vi "Show UI.vi"(0 "reference in":refnum<class "UI Manager Proxy.lvclass">, 2 "UI Type":T1, 5 "Error In":errorcluster) -> (14 "reference out":refnum<class "UI Manager Proxy.lvclass">, 19 "Error Out":errorcluster)   [LabVIEW 2024, in "UI Manager Proxy.lvclass"]
uses:
  UI Manager Proxy.lvclass
  UIType.ctl
  UI Manager_class/UI Manager.lvclass
  UI Manager Proxy.lvclass/UI Manager Proxy.ctl
panel:
  # "Connector Pane"
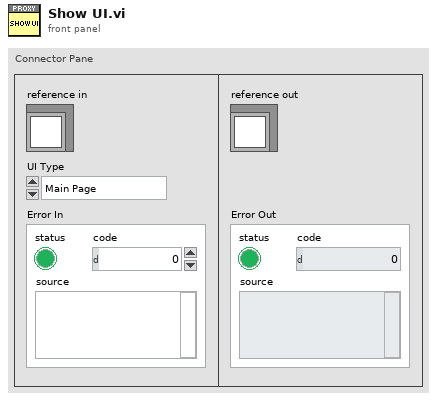
[diagram p1: front panel]
types:
  T1 = typedef "UIType.ctl" = enum16{"Main Page", "Settings Page", "Debugging Page"}
  T2 = typedef "UI Manager Proxy.lvclass/ObjectAttributes.ctl" = cluster{"UI Manager":refnum<class "UI Manager.lvclass">, "UserLevel":T3}
  T3 = typedef "UserLevel.ctl" = enum16{"System Manager", "Admin", "Operator"}
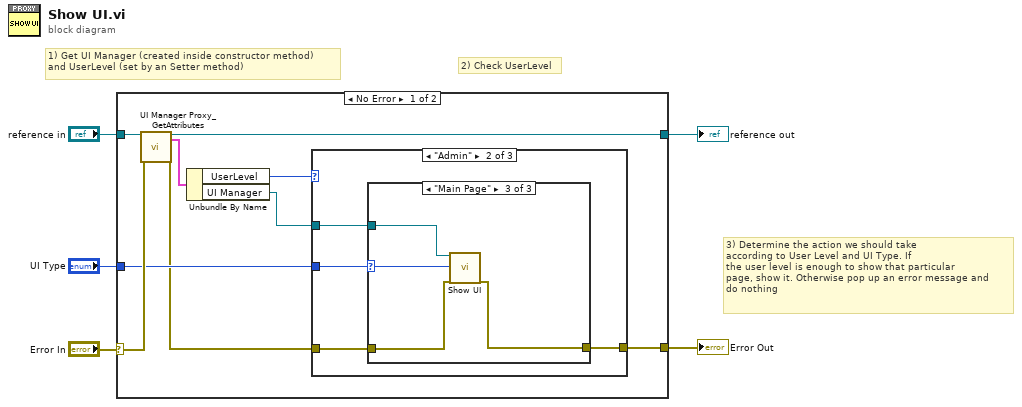
[diagram p0: block diagram]
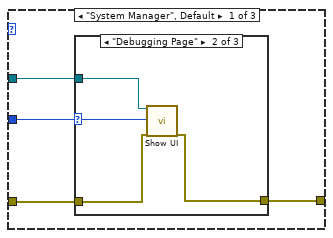
[diagram p2: hidden frame]
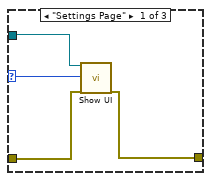
[diagram p3: hidden frame]
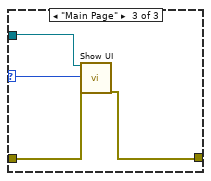
[diagram p4: hidden frame]
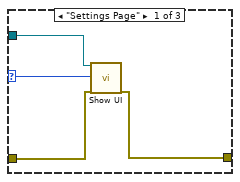
[diagram p5: hidden frame]
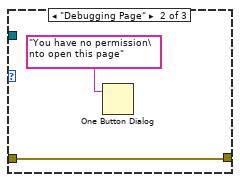
[diagram p6: hidden frame]
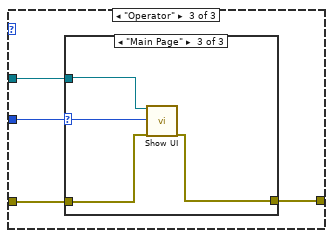
[diagram p7: hidden frame]
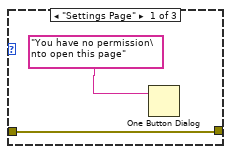
[diagram p8: hidden frame]
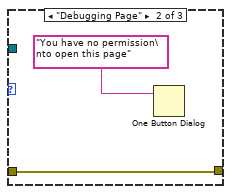
[diagram p9: hidden frame]
diagram:
  # "3) Determine the action we should take\naccording to User Level and UI Type. If\nthe user level is enough to show that particular\npage, show it. Otherwise pop up an error message and\ndo nothing"
  # "2) Check UserLevel"
  # "1) Get UI Manager (created inside constructor method) \nand UserLevel (set by an Setter method)"
  n1 = case shown="No Error" "Error In" {
    selector: "Error In" -> [w14 w58]
    tunnel: [w7 w58] -> w4
    tunnel: [w11 w57] -> w2
    tunnel: "reference in" -> [w12 w57]
    tunnel: "UI Type" -> [w9 _]
    frame No Error {
      n2 = call "UI Manager Proxy_GetAttributes.vi"("reference in"=w12, "Error In"=w14) -> ("reference out"=w11:refnum<class "UI Manager Proxy.lvclass">, "Data"=w13:T2, "Error Out"=w8:errorcluster)  [unwired: 14 in, 1 out]
      n3 = Unbundle By Name(w13) -> ("UserLevel"=w10:T3, "UI Manager"=w6:refnum<class "UI Manager.lvclass">)
      n4 = case shown="\"Admin\"" w10 {
        tunnel: w9 -> [w18 w34 w48]
        tunnel: w8 -> [w17 w33 w47]
        tunnel: [w16 w32 w46] -> w7
        tunnel: w6 -> [w15 w31 w45]
        frame "System Manager", Default {
          n5 = case shown="\"Debugging Page\"" w18 {
            selector: w18 -> [w22 w26 w30]
            tunnel: w17 -> [w21 w25 w28]
            tunnel: [w20 w24 w29] -> w16
            tunnel: w15 -> [w19 w23 w27]
            frame "Settings Page" {
              n6 = call-dynamic "Show UI.vi"("reference in"=w19, "UI Type"=w22, "Error In"=w21) -> ("Error Out"=w20:errorcluster)  [unwired: 15 in, 1 out]
            }
            frame "Debugging Page" {
              n7 = call-dynamic "Show UI.vi"("reference in"=w23, "UI Type"=w26, "Error In"=w25) -> ("Error Out"=w24:errorcluster)  [unwired: 15 in, 1 out]
            }
            frame "Main Page" {
              n8 = call-dynamic "Show UI.vi"("reference in"=w27, "UI Type"=w30, "Error In"=w28) -> ("Error Out"=w29:errorcluster)  [unwired: 15 in, 1 out]
            }
          }
        }
        frame "Admin" {
          n9 = case shown="\"Main Page\"" w34 {
            selector: w34 -> [w38 _ w44]
            tunnel: w33 -> [w36 w39 w43]
            tunnel: [w37 w39 w42] -> w32
            tunnel: w31 -> [w35 _ w41]
            frame "Settings Page" {
              n10 = call-dynamic "Show UI.vi"("reference in"=w35, "UI Type"=w38, "Error In"=w36) -> ("Error Out"=w37:errorcluster)  [unwired: 15 in, 1 out]
            }
            frame "Debugging Page" {
              n11 = One Button Dialog(message="You have no permission\nto open this page") -> ()  [unwired: 1 in, 1 out]
            }
            frame "Main Page" {
              n12 = call-dynamic "Show UI.vi"("reference in"=w41, "UI Type"=w44, "Error In"=w43) -> ("Error Out"=w42:errorcluster)  [unwired: 15 in, 1 out]
            }
          }
        }
        frame "Operator" {
          n13 = case shown="\"Main Page\"" w48 {
            selector: w48 -> [_ _ w56]
            tunnel: w47 -> [w49 w51 w55]
            tunnel: [w49 w51 w54] -> w46
            tunnel: w45 -> [_ _ w53]
            frame "Settings Page" {
              n14 = One Button Dialog(message="You have no permission\nto open this page") -> ()  [unwired: 1 in, 1 out]
            }
            frame "Debugging Page" {
              n15 = One Button Dialog(message="You have no permission\nto open this page") -> ()  [unwired: 1 in, 1 out]
            }
            frame "Main Page" {
              n16 = call-dynamic "Show UI.vi"("reference in"=w53, "UI Type"=w56, "Error In"=w55) -> ("Error Out"=w54:errorcluster)  [unwired: 15 in, 1 out]
            }
          }
        }
      }
    }
    frame Error {
    }
  }
  "Error Out" <- w4
  "reference out" <- w2
